vi "SDG60ConfBurst.vi"(0 "VISA resource name in":refnum<visa-resource-name>="USB0::0xF4EC::0x1101::SDG6XEBC5R0119::INSTR", 1 "Channel (1:Channel 1)":i32(ring)=1 items=["Channel 1"=1, "Channel 2"=2], 2 "Enable Burst Mode (T:Enable)":bool=TRUE, 3 "Trigger Source (0: Internal)":u16(ring) items=["Internal", "External", "Manual"], 4 "Burst Cycle (0: N-Cycle)":u16(ring) items=["N-Cycle", "Infinite"], 5 "Burst Delay (1.352 us)":dbl=1.352e-06, 6 "Burst Period (0.01 s)":dbl=0.01 format="%#.3g", 7 "error in (no error)":errorcluster, 8 "Triggered/Gated: (0:Triggered)":u16(ring) items=["Triggered", "Gated"], 9 "Trigger Out Mode (0: Off)":u16(ring) items=["Off", "Rise", "Fall"], 10 "Gate Polarity 0: Positive":u16(ring) items=["Positive", "Negative"], 11 "Start Phase (0.0 degrees)":dbl=0.002 min=0.0 max=360.0 format="%#.15g", 12 "Number of Cycles":i32=1, 13 "External Trigger Condition (0: Rise)":u16(ring) items=["Rise", "Fall"]) -> (20 "VISA resource name out":refnum<visa-resource-name>, 27 "error out":errorcluster)   [LabVIEW 2018]
doc: "Configures and enables burst output mode.\n\nNote: Burst mode is not available for noise waveform."
panel:
  # "Can't have manual trigger on gated"
  # "Resolution: 0.1degrees"
  # "Range: 1.352us-100s\n6 digits precision"
  # "Trigger values can't be changed\nTrigger High: 2-5.5V\nTrigger Low: -0.5-0.8V"
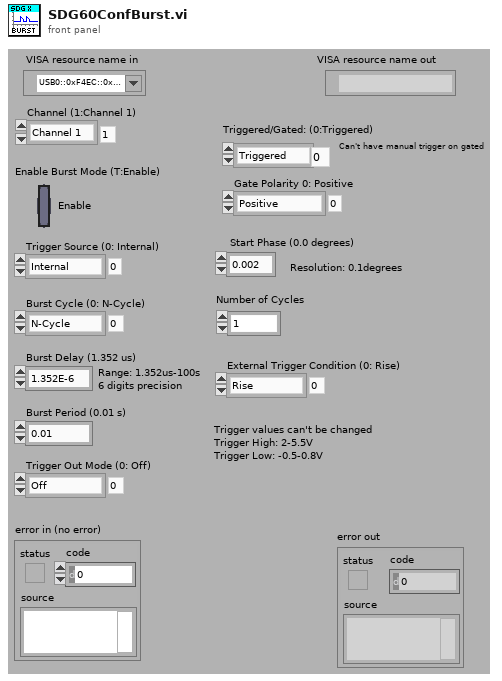
[diagram p1: front panel]
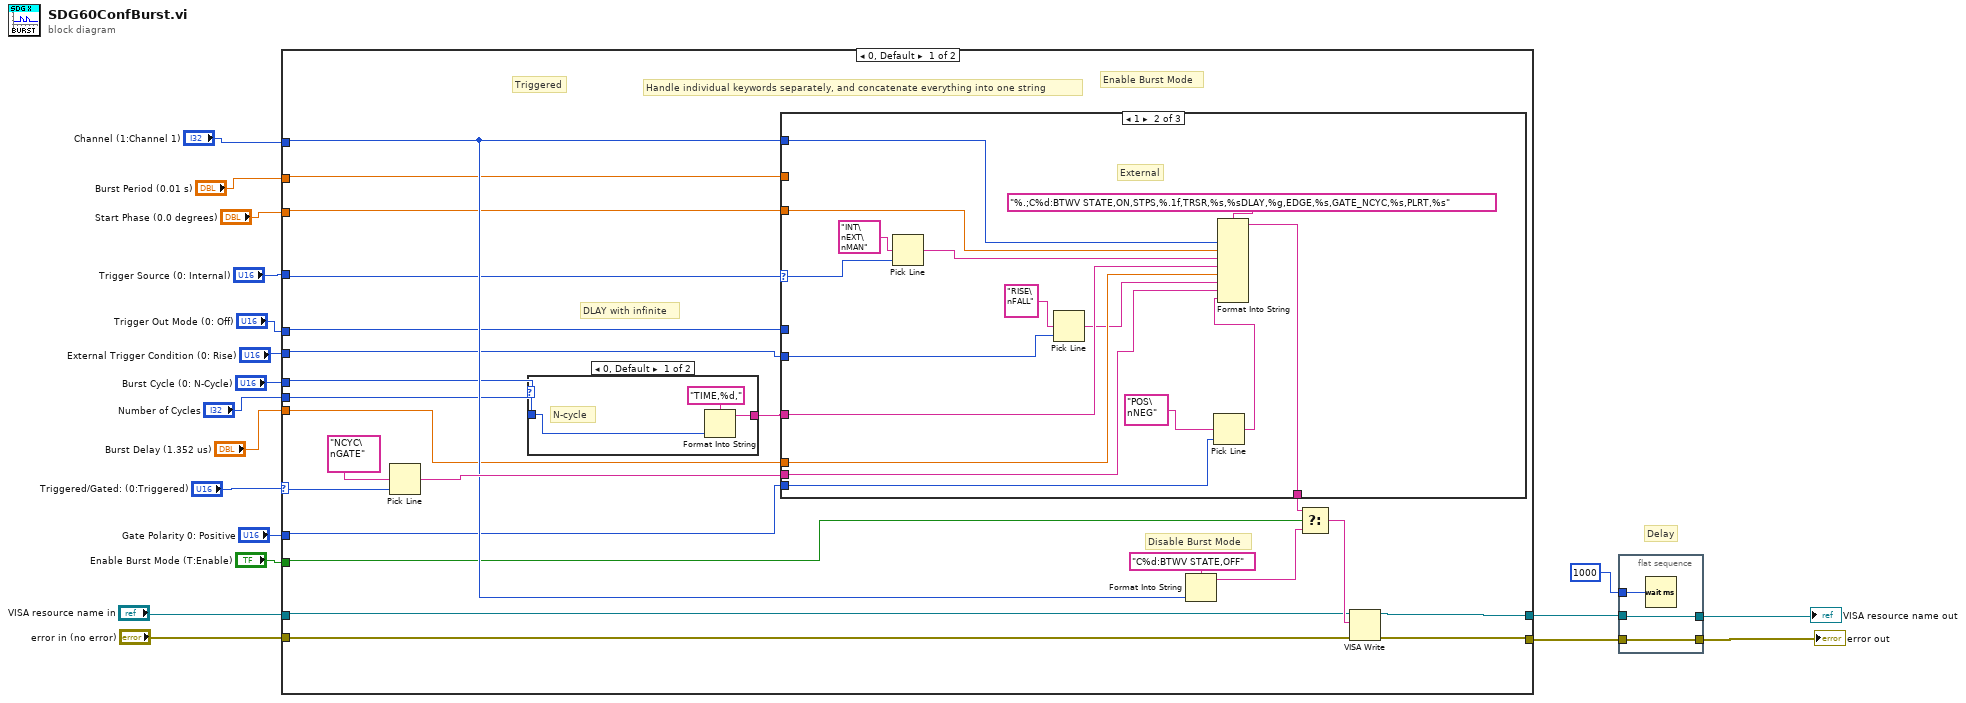
[diagram p0: block diagram]
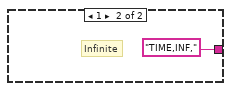
[diagram p2: hidden frame]
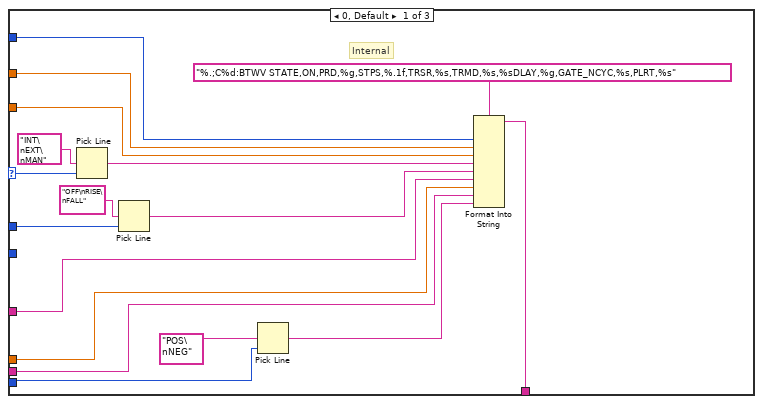
[diagram p3: hidden frame]
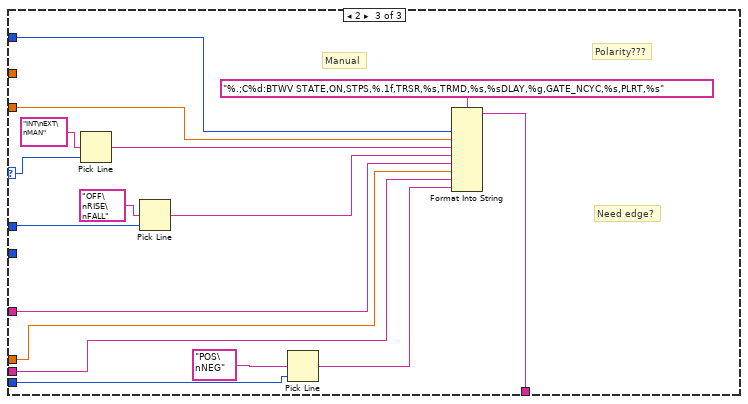
[diagram p4: hidden frame]
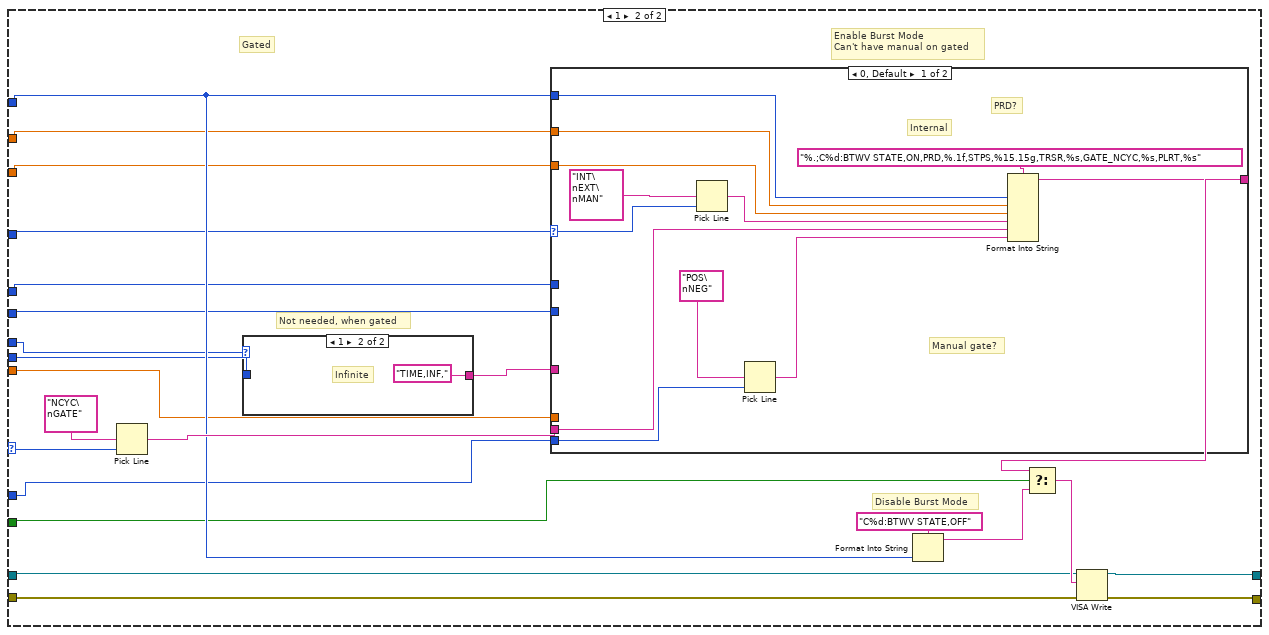
[diagram p5: hidden frame]
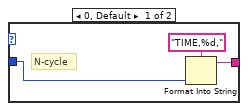
[diagram p6: hidden frame]
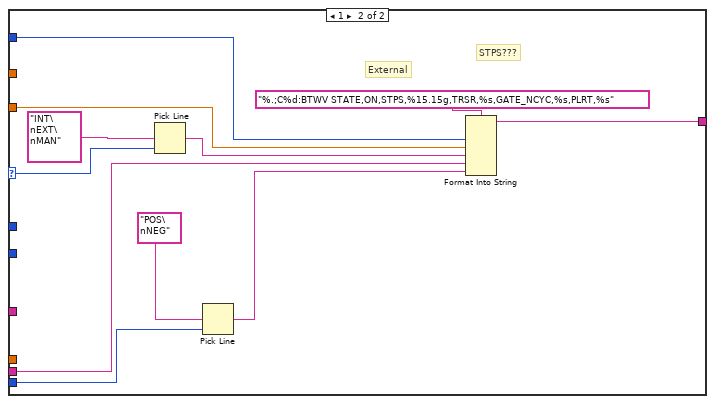
[diagram p7: hidden frame]
diagram:
  # "Delay"
  n1 = case shown="0, Default" "Triggered/Gated: (0:Triggered)" {
    selector: "Triggered/Gated: (0:Triggered)" -> [w27 w104]
    tunnel: "VISA resource name in" -> [w24 w101]
    tunnel: "error in (no error)" -> [w23 w100]
    tunnel: [w21 w98] -> w16
    tunnel: [w22 w99] -> w14
    tunnel: "Channel (1:Channel 1)" -> [w35 w112]
    tunnel: "Burst Cycle (0: N-Cycle)" -> [w29 w106]
    tunnel: "Burst Period (0.01 s)" -> [w34 w111]
    tunnel: "Start Phase (0.0 degrees)" -> [w33 w110]
    tunnel: "Trigger Source (0: Internal)" -> [w32 w109]
    tunnel: "Trigger Out Mode (0: Off)" -> [w31 w108]
    tunnel: "External Trigger Condition (0: Rise)" -> [w30 w107]
    tunnel: "Enable Burst Mode (T:Enable)" -> [w25 w102]
    tunnel: "Gate Polarity 0: Positive" -> [w26 w103]
    tunnel: "Burst Delay (1.352 us)" -> [w28 w105]
    tunnel: "Number of Cycles" -> [w20 w97]
    frame 0, Default {
      # "Handle individual keywords separately, and concatenate everything into one string"
      # "DLAY with infinite"
      # "Disable Burst Mode"
      # "Enable Burst Mode"
      # "Triggered"
      n2 = Pick Line(multi-line string="NCYC\nGATE", line index=w27) -> (output string=w42:string)  [unwired: 1 in]
      n3 = case shown="0, Default" w29 {
        tunnel: [w44 "TIME,INF,"] -> w38
        tunnel: w20 -> [w43 _]
        frame 0, Default {
          # "N-cycle"
          n4 = Format Into String(format string="TIME,%d,", w43) -> (resulting string=w44:string)  [unwired: 2 in, 1 out]
        }
        frame 1 {
          # "Infinite"
        }
      }
      n5 = case shown="1" w32 {
        selector: w32 -> [w60 w75 w92]
        tunnel: w35 -> [w61 w77 w93]
        tunnel: w28 -> [w49 w71 w83]
        tunnel: [w56 w69 w89] -> w39
        tunnel: w31 -> [w55 _ w90]
        tunnel: w33 -> [w54 w76 w88]
        tunnel: w38 -> [w51 w72 w85]
        tunnel: w34 -> [w53 _ _]
        tunnel: w30 -> [_ w68 _]
        tunnel: w26 -> [w50 w66 w82]
        tunnel: w42 -> [w47 w64 w80]
        frame 0, Default {
          # "Internal"
          n6 = Pick Line(multi-line string="INT\nEXT\nMAN", line index=w60) -> (output string=w58:string)  [unwired: 1 in]
          n7 = Pick Line(multi-line string="OFF\nRISE\nFALL", line index=w55) -> (output string=w57:string)  [unwired: 1 in]
          n8 = Pick Line(multi-line string="POS\nNEG", line index=w50) -> (output string=w48:string)  [unwired: 1 in]
          n9 = Format Into String(format string="%.;C%d:BTWV STATE,ON,PRD,%g,STPS,%.1f,TRSR,%s,TRMD,%s,%sDLAY,%g,GATE_NCYC,%s,PLRT,%s", w61, w53, w54, w58, w57, w51, w49, w47, w48) -> (resulting string=w56:string)  [unwired: 2 in, 1 out]
        }
        frame 1 {
          # "External"
          n10 = Pick Line(multi-line string="INT\nEXT\nMAN", line index=w75) -> (output string=w73:string)  [unwired: 1 in]
          n11 = Pick Line(multi-line string="RISE\nFALL", line index=w68) -> (output string=w70:string)  [unwired: 1 in]
          n12 = Pick Line(multi-line string="POS\nNEG", line index=w66) -> (output string=w65:string)  [unwired: 1 in]
          n13 = Format Into String(format string="%.;C%d:BTWV STATE,ON,STPS,%.1f,TRSR,%s,%sDLAY,%g,EDGE,%s,GATE_NCYC,%s,PLRT,%s", w77, w76, w73, w72, w71, w70, w64, w65) -> (resulting string=w69:string)  [unwired: 2 in, 1 out]
        }
        frame 2 {
          # "Need edge?"
          # "Polarity???"
          # "Manual"
          n14 = Pick Line(multi-line string="INT\nEXT\nMAN", line index=w92) -> (output string=w87:string)  [unwired: 1 in]
          n15 = Pick Line(multi-line string="OFF\nRISE\nFALL", line index=w90) -> (output string=w86:string)  [unwired: 1 in]
          n16 = Pick Line(multi-line string="POS\nNEG", line index=w82) -> (output string=w81:string)  [unwired: 1 in]
          n17 = Format Into String(format string="%.;C%d:BTWV STATE,ON,STPS,%.1f,TRSR,%s,TRMD,%s,%sDLAY,%g,GATE_NCYC,%s,PLRT,%s", w93, w88, w87, w86, w85, w83, w80, w81) -> (resulting string=w89:string)  [unwired: 2 in, 1 out]
        }
      }
      n18 = Format Into String(format string="C%d:BTWV STATE,OFF", w35) -> (resulting string=w40:string)  [unwired: 2 in, 1 out]
      n19 = Select(t=w39, s=w25, f=w40) -> (s? t:f=w41:string)
      n20 = VISA Write(VISA resource name=w24, write buffer=w41, error in (no error)=w23) -> (VISA resource name out=w22:refnum<visa-resource-name>, error out=w21:errorcluster)  [unwired: 1 out]
    }
    frame 1 {
      # "Not needed, when gated"
      # "Disable Burst Mode"
      # "Enable Burst Mode\nCan't have manual on gated"
      # "Gated"
      n21 = Pick Line(multi-line string="NCYC\nGATE", line index=w104) -> (output string=w118:string)  [unwired: 1 in]
      n22 = case shown="1" w106 {
        tunnel: [w120 "TIME,INF,"] -> w115
        tunnel: w97 -> [w119 _]
        frame 0, Default {
          # "N-cycle"
          n23 = Format Into String(format string="TIME,%d,", w119) -> (resulting string=w120:string)  [unwired: 2 in, 1 out]
        }
        frame 1 {
          # "Infinite"
        }
      }
      n24 = case shown="0, Default" w109 {
        selector: w109 -> [w132 w142]
        tunnel: w112 -> [w133 w144]
        tunnel: w105 -> [_ _]
        tunnel: w108 -> [_ _]
        tunnel: w110 -> [w124 w143]
        tunnel: w115 -> [_ _]
        tunnel: w111 -> [w123 _]
        tunnel: w107 -> [_ _]
        tunnel: w103 -> [w128 w138]
        tunnel: w118 -> [w126 w136]
        tunnel: [w125 w135] -> w96
        frame 0, Default {
          # "Manual gate?"
          # "PRD?"
          # "Internal"
          n25 = Pick Line(multi-line string="INT\nEXT\nMAN", line index=w132) -> (output string=w130:string)  [unwired: 1 in]
          n26 = Pick Line(multi-line string="POS\nNEG", line index=w128) -> (output string=w127:string)  [unwired: 1 in]
          n27 = Format Into String(format string="%.;C%d:BTWV STATE,ON,PRD,%.1f,STPS,%15.15g,TRSR,%s,GATE_NCYC,%s,PLRT,%s", w133, w123, w124, w130, w126, w127) -> (resulting string=w125:string)  [unwired: 2 in, 1 out]
        }
        frame 1 {
          # "STPS???"
          # "External"
          n28 = Pick Line(multi-line string="INT\nEXT\nMAN", line index=w142) -> (output string=w140:string)  [unwired: 1 in]
          n29 = Pick Line(multi-line string="POS\nNEG", line index=w138) -> (output string=w137:string)  [unwired: 1 in]
          n30 = Format Into String(format string="%.;C%d:BTWV STATE,ON,STPS,%15.15g,TRSR,%s,GATE_NCYC,%s,PLRT,%s", w144, w143, w140, w136, w137) -> (resulting string=w135:string)  [unwired: 2 in, 1 out]
        }
      }
      n31 = Format Into String(format string="C%d:BTWV STATE,OFF", w112) -> (resulting string=w116:string)  [unwired: 2 in, 1 out]
      n32 = Select(t=w96, s=w102, f=w116) -> (s? t:f=w117:string)
      n33 = VISA Write(VISA resource name=w101, write buffer=w117, error in (no error)=w100) -> (VISA resource name out=w99:refnum<visa-resource-name>, error out=w98:errorcluster)  [unwired: 1 out]
    }
  }
  n34 = flat-sequence {
    tunnel: w16 -> [w148]
    tunnel: [w148] -> w13
    tunnel: u32 1000 ("Delay Time (10)") -> [w147]
    tunnel: w14 -> [w146]
    tunnel: [w146] -> w12
    frame #0 {
      n35 = Wait (ms)(milliseconds to wait=w147) -> ()  [unwired: 1 out]
    }
  }
  "error out" <- w13
  "VISA resource name out" <- w12
